vi "drawwinlose.vi"(9 "new picture in":picture, 10 "win":bool, 11 "lose":bool) -> (3 "new picture out":picture)   [LabVIEW 2025]
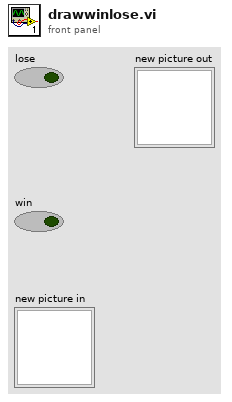
[diagram p1: front panel]
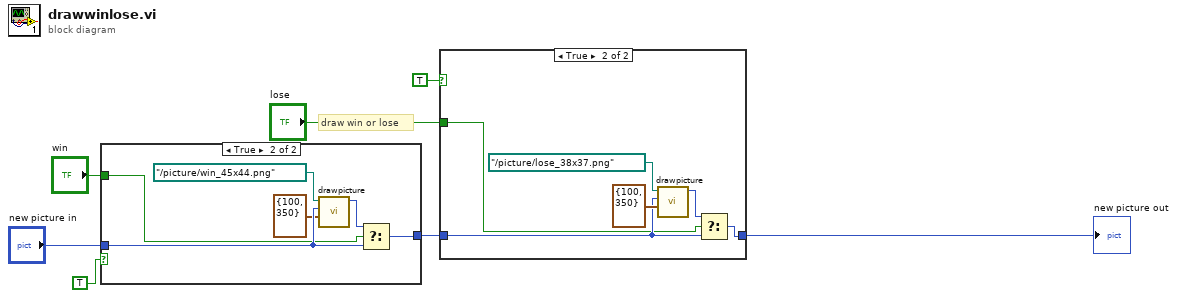
[diagram p0: block diagram]
diagram:
  # "draw win or lose"
  n1 = case shown="True" TRUE {
    tunnel: "new picture in" -> [w8 w13]
    tunnel: [w8 w11] -> w4
    tunnel: "win" -> [_ w9]
    frame False {
    }
    frame True {
      n2 = call "drawpicture.vi"("y"=cluster{"left":i16, "top":i16} {"left"=100, "top"=350}, "2D Picture"=w13, "name or relative path"=path "../picture/win_45x44.png") -> ("new picture"=w12:picture)  [unwired: 8 in]
      n3 = Select(t=w12, s=w9, f=w13) -> (s? t:f=w11:picture)
    }
  }
  n4 = case shown="True" TRUE {
    tunnel: w4 -> [w15 w18]
    tunnel: [w15 w17] -> w5
    tunnel: "lose" -> [_ w16]
    frame False {
    }
    frame True {
      n5 = call "drawpicture.vi"("y"=cluster{"left":i16, "top":i16} {"left"=100, "top"=350}, "2D Picture"=w18, "name or relative path"=path "../picture/lose_38x37.png") -> ("new picture"=w20:picture)  [unwired: 8 in]
      n6 = Select(t=w20, s=w16, f=w18) -> (s? t:f=w17:picture)
    }
  }
  "new picture out" <- w5
